vi "Catch.vi"(8 "error in (no error)":errorcluster) -> (0 "error out":errorcluster, 3 "Error out":refnum<class "Error.lvclass">)   [LabVIEW 2022 SP3, in "Error.lvlib" / "Error.lvclass"]
uses:
  Error.lvclass
  NoError/NoError.lvclass
  C:/Users/jakub/repos/gh/lv-error/Source/Error/Error/Error.lvclass
  Error.lvclass/Error.ctl
  <vilib>/Utility/error.llb/Trim Whitespace One-Sided.vi
  <vilib>/regexp/Match Regular Expression.xnode
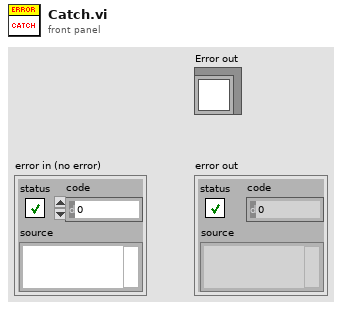
[diagram p1: front panel]
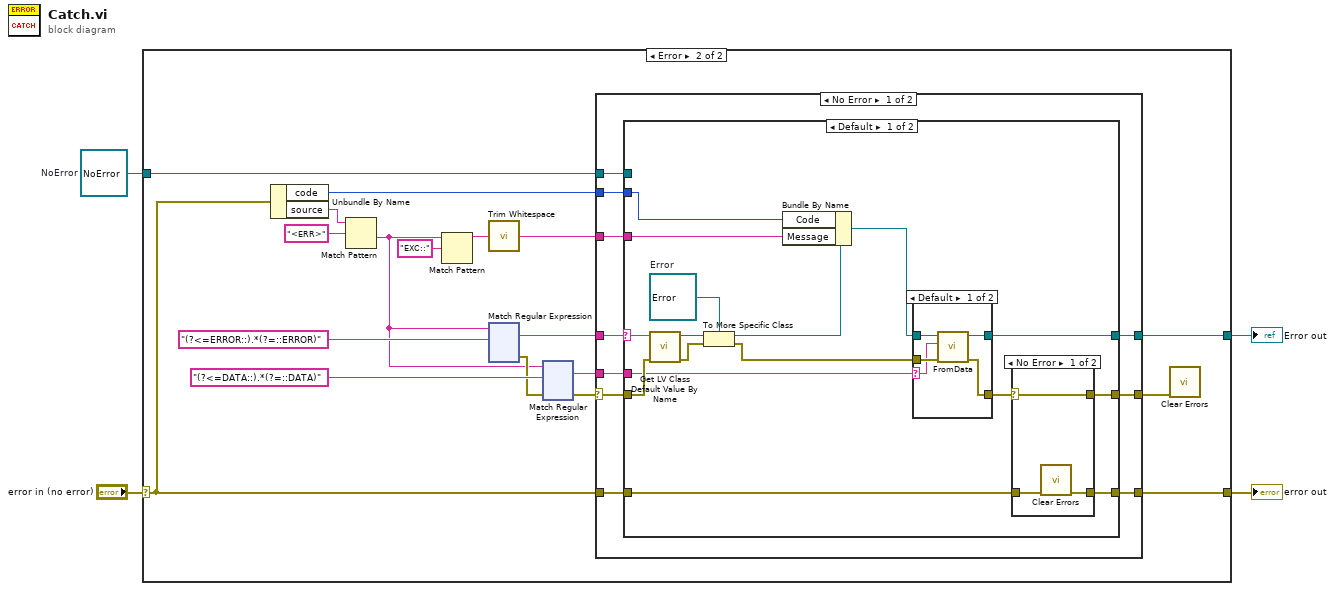
[diagram p0: block diagram]
diagram:
  w1 = refnum<class "NoError.lvclass"> refnum  # NoError
  n1 = case shown="Error" "error in (no error)" {
    selector: "error in (no error)" -> [w6 w8]
    tunnel: [w6 w7] -> w3
    tunnel: [w5 w17] -> w2
    tunnel: w1 -> [w5 w16]
    frame No Error {
    }
    frame Error {
      n2 = Unbundle By Name(w8) -> ("code"=w15:i32, "source"=w14:string)
      n3 = Match Pattern(string=w14, regular expression="<ERR>") -> (after substring=w12:string)  [unwired: 1 in, 3 out]
      n4 = Match Pattern(string=w12, regular expression="EXC::") -> (before substring=w10:string)  [unwired: 1 in, 3 out]
      n5 = call <vilib>:"Trim Whitespace.vi"("string"=w10) -> ("trimmed string"=w9:string)  [unwired: 1 in]
      n6 = xnode "Match Regular Expression"("input string"=w12, "regular expression"="(?<=ERROR::).*(?=::ERROR)") -> ("whole match"=w20:string, "error out"=w22:errorcluster)  [unwired: 4 in, 3 out]
      n7 = xnode "Match Regular Expression"("input string"=w12, "regular expression"="(?<=DATA::).*(?=::DATA)", "error in"=w22) -> ("whole match"=w19:string, "error out"=w21:errorcluster)  [unwired: 3 in, 3 out]
      n8 = case shown="No Error" w21 {
        selector: w21 -> [w33 w68]
        tunnel: w20 -> [w34 _]
        tunnel: w19 -> [w32 _]
        tunnel: [w31 w68] -> w18
        tunnel: [w29 w67] -> w17
        tunnel: w16 -> [w30 w67]
        tunnel: w15 -> [w28 _]
        tunnel: w9 -> [w27 _]
        tunnel: w8 -> [w26 w66]
        tunnel: [w25 w66] -> w7
        frame No Error {
          n9 = case shown="Default" w34 {
            selector: w34 -> [w50 _]
            tunnel: w33 -> [w49 w65]
            tunnel: w32 -> [w47 _]
            tunnel: [w37 w65] -> w31
            tunnel: [w43 w64] -> w29
            tunnel: w30 -> [_ w64]
            tunnel: w28 -> [w40 _]
            tunnel: w27 -> [w39 _]
            tunnel: w26 -> [w36 w63]
            tunnel: [w35 w63] -> w25
            frame Default {
              w44 = refnum<class "Error.lvclass"> refnum  # Error
              n10 = call <vilib>:"Get LV Class Default Value By Name.vi"("error in (no error)"=w49, "class name"=w50) -> ("error out"=w46:errorcluster, "object"=w48:refnum<class>)  [unwired: 8 in]
              n11 = To More Specific Class(target class=w44, reference=w48, error in=w46) -> (specific class reference=w42:refnum<class "Error.lvclass">, error out=w45:errorcluster)
              n12 = Bundle By Name(cluster=w42, "Code"=w40, "Message"=w39) -> (w41:refnum<class "Error.lvclass">)
              n13 = case shown="Default" w47 {
                selector: w47 -> [w58 _]
                tunnel: w45 -> [w60 w62]
                tunnel: w41 -> [w57 w61]
                tunnel: [w59 w62] -> w38
                tunnel: [w56 w61] -> w43
                frame Default {
                  n14 = call-dynamic "FromData.vi"("error in (no error)"=w60, "Data"=w58, "Error in"=w57) -> ("error out"=w59:errorcluster, "Error out"=w56:refnum<class "Error.lvclass">)  [unwired: 7 in]
                }
                frame "" {
                }
              }
              n15 = case shown="No Error" w38 {
                selector: w38 -> [w53 w55]
                tunnel: [w53 w55] -> w37
                tunnel: w36 -> [w52 w54]
                tunnel: [w51 w54] -> w35
                frame No Error {
                  n16 = call <vilib>:"Clear Errors.vi"("error in (no error)"=w52) -> ("error out"=w51:errorcluster)  [unwired: 5 in, 1 out]
                }
                frame Error {
                }
              }
            }
            frame "" {
            }
          }
        }
        frame Error {
        }
      }
      n17 = call <vilib>:"Clear Errors.vi"("error in (no error)"=w18) -> ()  [unwired: 5 in, 2 out]
    }
  }
  "error out" <- w3
  "Error out" <- w2
